vi "Open Project.vi"(7 "Open Project Window ?":bool, 8 "error in (no error)":errorcluster, 10 "Project Path in":path, 11 "Application in":refnum<vi>) -> (0 "error out":errorcluster, 2 "Project out":refnum<vi>, 3 "Application out":refnum<vi>)   [LabVIEW 2019, in "VI Scripting Tools.lvlib"]
uses:
  VI Scripting Tools.lvlib
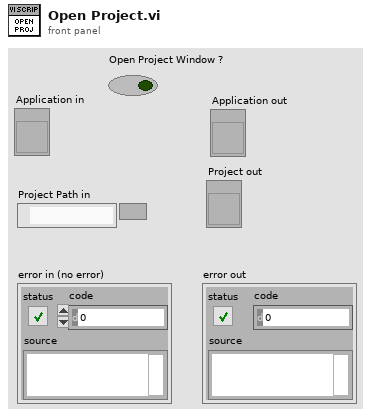
[diagram p1: front panel]
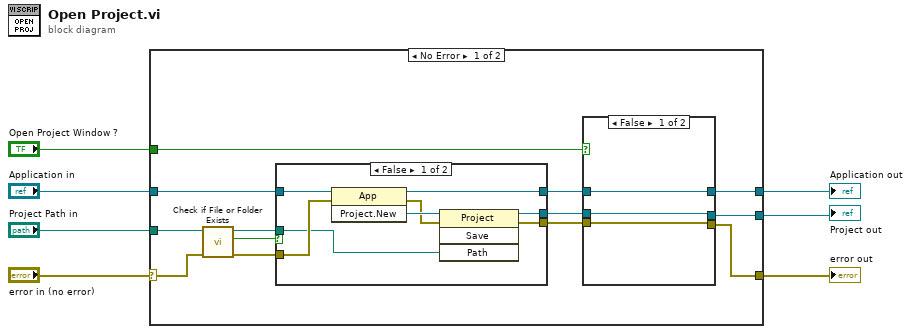
[diagram p0: block diagram]
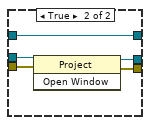
[diagram p2: hidden frame]
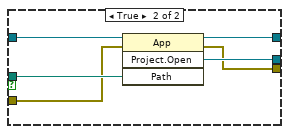
[diagram p3: hidden frame]
diagram:
  n1 = case shown="No Error" "error in (no error)" {
    selector: "error in (no error)" -> [w11 w44]
    tunnel: "Project Path in" -> [w20 _]
    tunnel: [w9 w43] -> w6
    tunnel: "Application in" -> [w16 w43]
    tunnel: "Open Project Window ?" -> [w8 _]
    tunnel: [w13 _] -> w3
    tunnel: [w12 w44] -> w2
    frame No Error {
      n2 = call <vilib>:"Check if File or Folder Exists.vi"("error in (no error)"=w11, "path"=w20) -> ("error out"=w17:errorcluster, "file or folder exists?"=w18:bool, "dup path"=w19:path)  [unwired: 7 in]
      n3 = case shown="False" w18 {
        tunnel: [w30 w38] -> w15
        tunnel: w19 -> [w31 w42]
        tunnel: w17 -> [w35 w40]
        tunnel: [w33 w41] -> w10
        tunnel: w16 -> [w32 w39]
        tunnel: [w29 w37] -> w14
        frame False {
          n4 = invoke class="App" method="Project.New"(reference=w32, error in=w35) -> (reference out=w33:refnum<vi>, error out=w34:errorcluster, "Project:New"=w36:refnum<vi>)  [unwired: 1 in]
          n5 = invoke class="Project" method="Save"(reference=w36, error in=w34, "Path"=w31) -> (reference out=w30:refnum<vi>, error out=w29:errorcluster)  [unwired: 1 in, 2 out]
        }
        frame True {
          n6 = invoke class="App" method="Project.Open"(reference=w39, error in=w40, "Path"=w42) -> (reference out=w41:refnum<vi>, error out=w37:errorcluster, "Project:Open"=w38:refnum<vi>)  [unwired: 1 in, 1 out]
        }
      }
      n7 = case shown="False" w8 {
        tunnel: w15 -> [w22 w28]
        tunnel: w14 -> [w21 w27]
        tunnel: [w22 w26] -> w13
        tunnel: [w21 w25] -> w12
        tunnel: w10 -> [w23 w24]
        tunnel: [w23 w24] -> w9
        frame False {
        }
        frame True {
          n8 = invoke class="Project" method="Open Window"(reference=w28, error in=w27) -> (reference out=w26:refnum<vi>, error out=w25:errorcluster)  [unwired: 1 in, 1 out]
        }
      }
    }
    frame Error {
    }
  }
  "Project out" <- w3
  "error out" <- w2
  "Application out" <- w6
